vi "Read_Write_Temp_Cluster.vi"(3 "Template Info Array":T3[](array[typedef]) {"Tolerance" min=0.0 format="%#.4f"}, 4 "Mode":T2, 5 "Template File":path) -> (0 "Template Info Array Out":T3[](array[typedef]) {"Tolerance" min=0.0 format="%#.4f"})   [LabVIEW 2016]
uses:
  File_Template_Clus.ctl
  Data plotting/subVIs/Dispose_Channel.ctl
  Controls/Global_mode.ctl
panel:
  in  "Dispose":T1
  # "> 20  or  <20  or  =hello   or \n£hello  (not equal to hello)"
  # "<<Characters_to_Match>>  <<Replace_Whole_String_with_this>>"
  # "<<Channel_Name>> contains <<Characters to match>> or\n<<Channel_Name>> does not contain <<Characters to match>>"
  # "<<Channel_Name_A>> + <<Channel_Name_B>> or\nConcatenate <<Channel_Name_A>> and <<Channel_Name_B>>"
  # "> 20  or  <20  or  =hello   or \n£hello  (not equal to hello)"
  # "<<Characters_to_Match>>  <<Replace_Whole_String_with_this>>"
  # "<<Channel_Name>> contains <<Characters to match>> or\n<<Channel_Name>> does not contain <<Characters to match>>"
  # "<<Channel_Name_A>> + <<Channel_Name_B>> or\nConcatenate <<Channel_Name_A>> and <<Channel_Name_B>>"
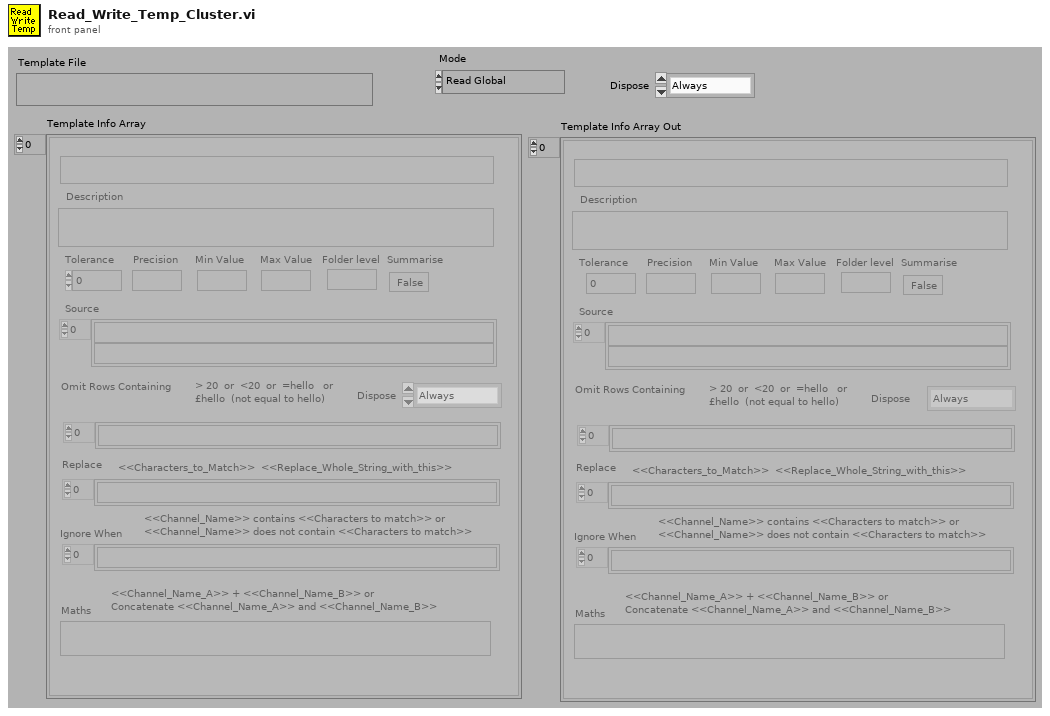
[diagram p1: front panel]
types:
  T1 = typedef "Dispose_Channel.ctl" = enum16{"Always", "If Blank", "Never"}
  T2 = typedef "Global_mode.ctl" = enum16{"Read Global", "Load Global From File", "Write Global to File"}
  T3 = typedef "File_Template_Clus.ctl" = cluster{"Template Channel Name":string, "Description":string, "Tolerance":dbl, "Precision":string, "Folder level":string, "Source":string[], "Replace":string[], "Summarise":bool, "Min Value":string, "Maths":string, "Omit Rows Containing":string[], "Ignore When":string[], "Max Value":string, "Dispose":T1}
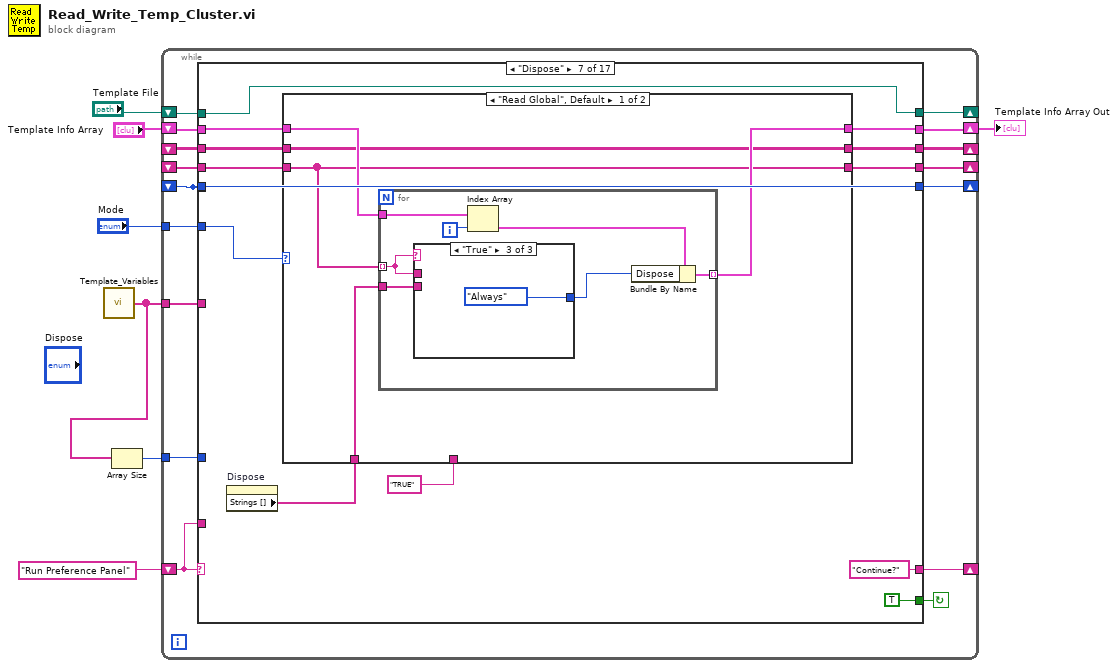
[diagram p0: block diagram]
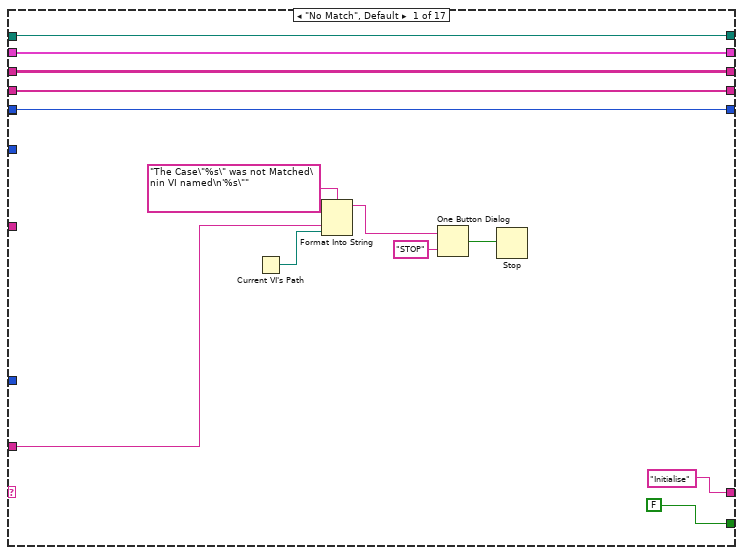
[diagram p2: hidden frame]
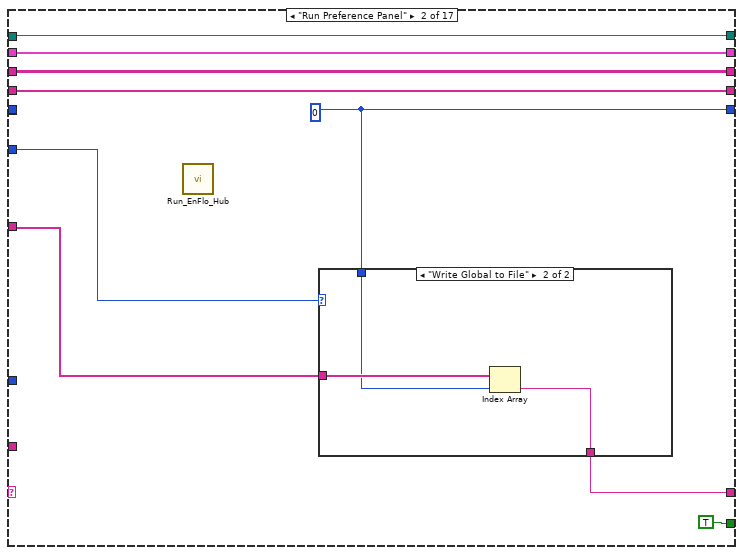
[diagram p3: hidden frame]
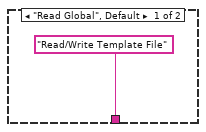
[diagram p4: hidden frame]
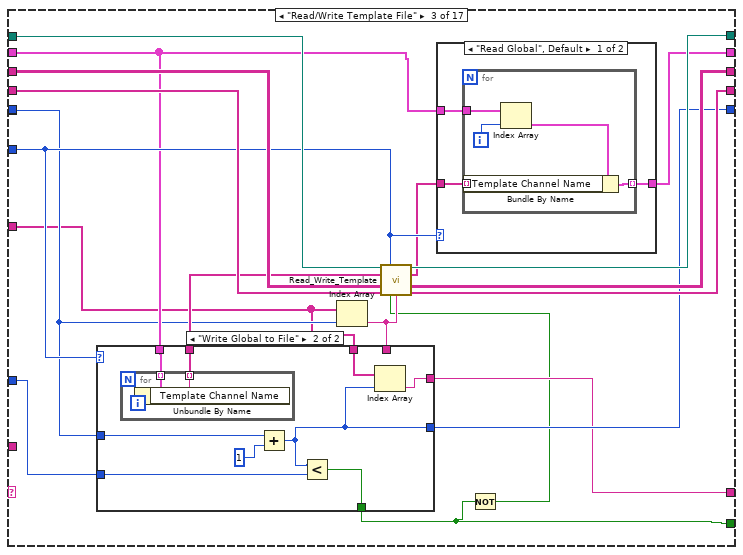
[diagram p5: hidden frame]
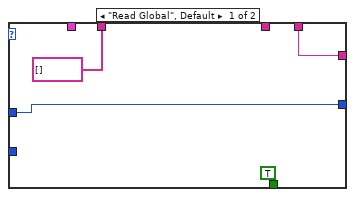
[diagram p7: hidden frame]
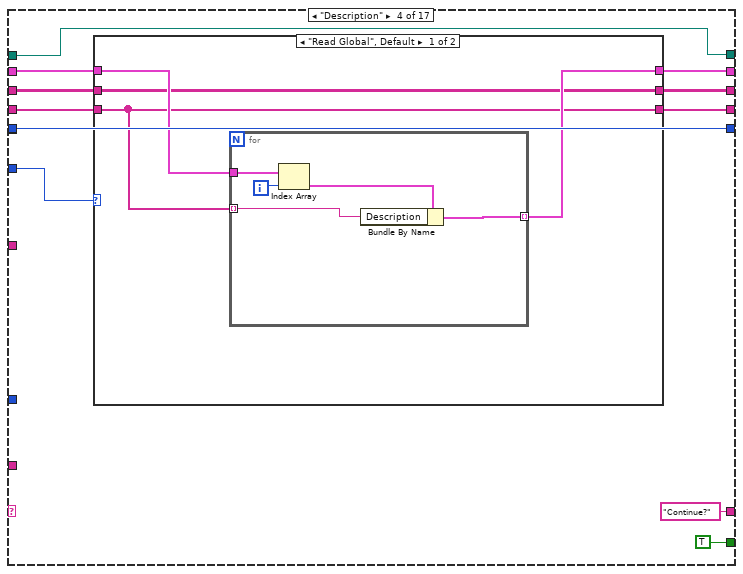
[diagram p8: hidden frame]
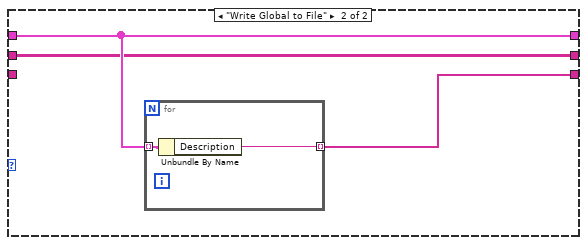
[diagram p9: hidden frame]
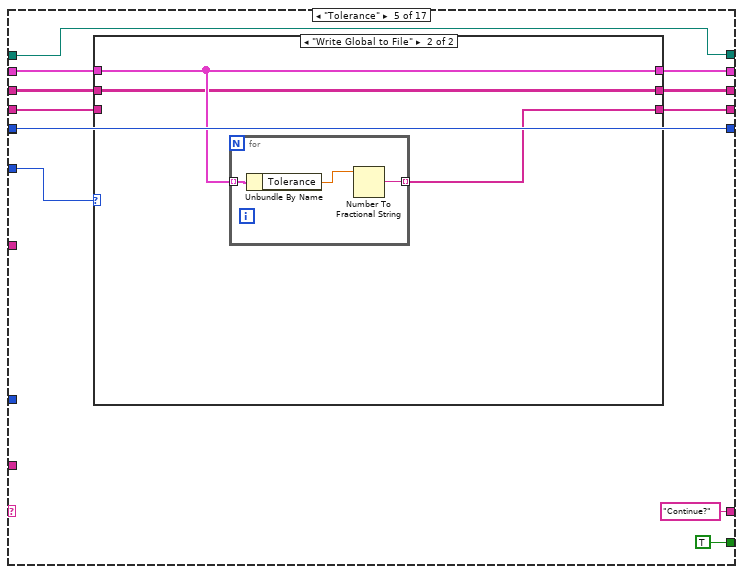
[diagram p10: hidden frame]
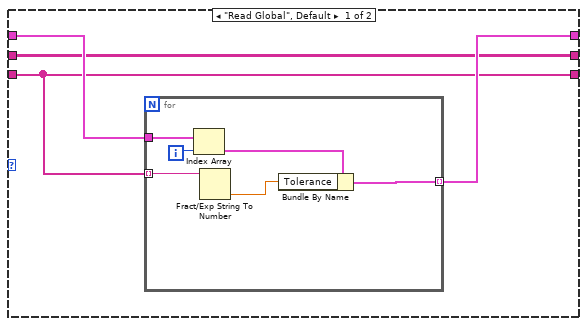
[diagram p11: hidden frame]
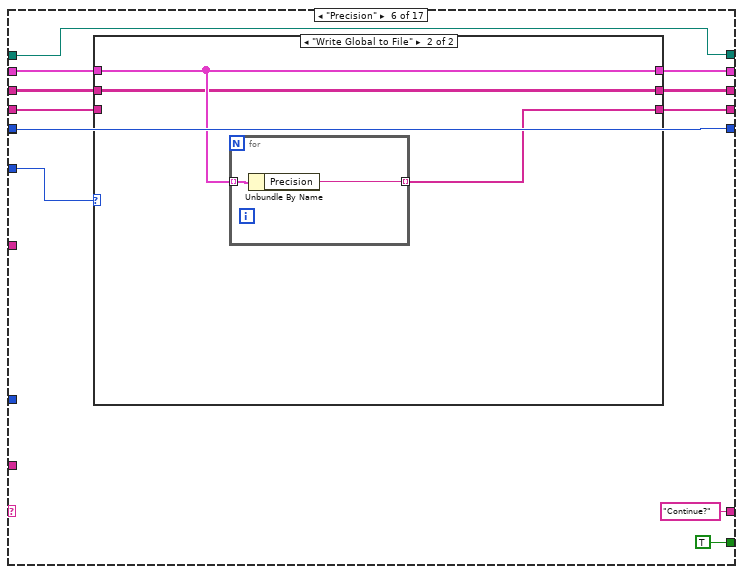
[diagram p12: hidden frame]
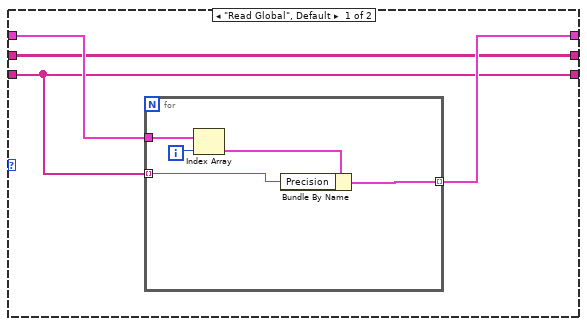
[diagram p13: hidden frame]
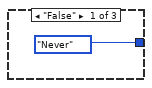
[diagram p14: hidden frame]
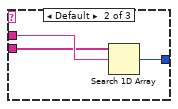
[diagram p15: hidden frame]
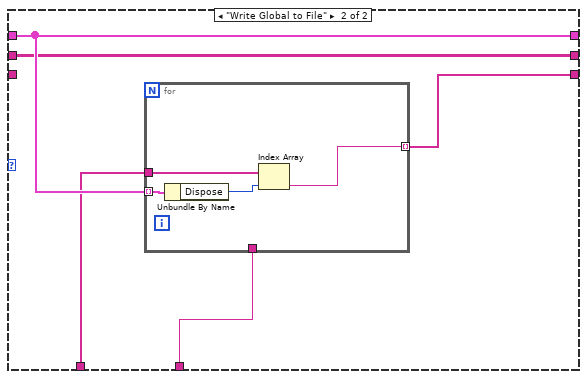
[diagram p16: hidden frame]
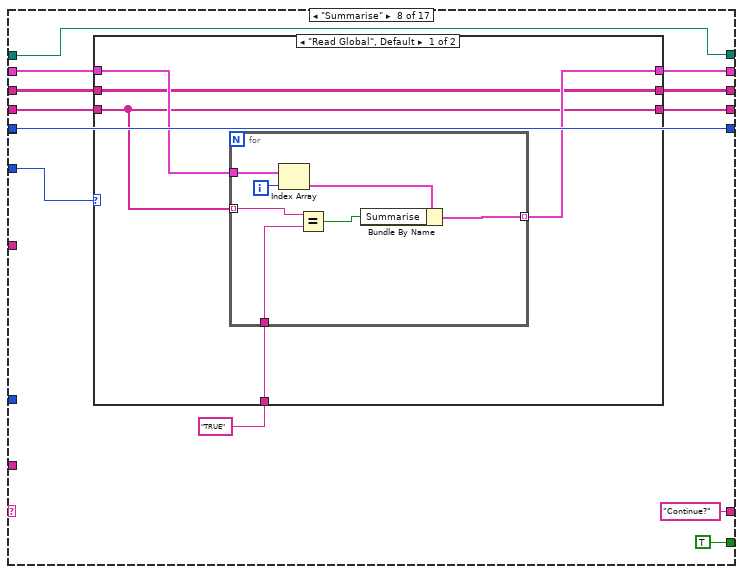
[diagram p17: hidden frame]
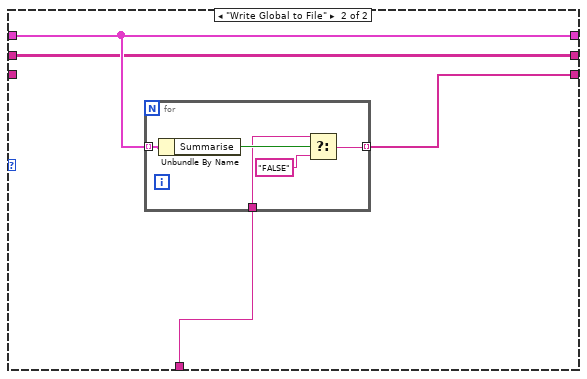
[diagram p18: hidden frame]
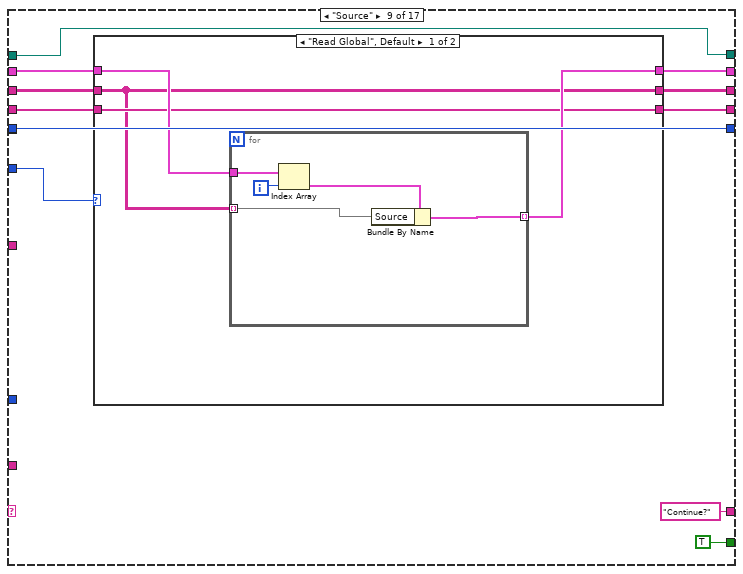
[diagram p19: hidden frame]
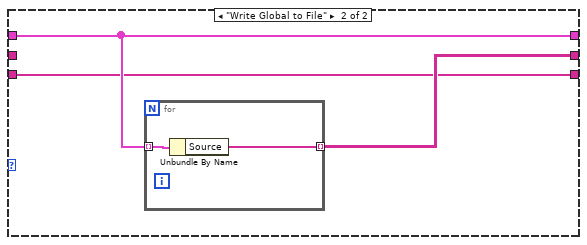
[diagram p20: hidden frame]
diagram:
  n1 = call "Template_Variables.vi"() -> ("Variable Names"=w1:string[])
  n2 = Array Size(array=w1) -> (size(s)=w2:i32)
  n3 = while {
    tunnel: w2 -> [w11]
    tunnel: "Mode" -> [w13]
    tunnel: w1 -> [w16]
    shift-left: "Template File" -> [w17]
    shift-right: [w8] -> _
    shift-left: _ -> [w10]
    shift-right: [w9] -> _
    shift-left: _ -> [w14]
    shift-right: [w18] -> _
    shift-left: _ -> [w15]
    shift-right: [w12] -> _
    shift-left: "Template Info Array" -> [w19]
    shift-right: [w20] -> w4
    shift-left: "Run Preference Panel" -> [w21]
    shift-right: [w22] -> _
    stop <- w23 continue-if-true
    n4 = case shown="\"Dispose\"" w21 {
      tunnel: [FALSE TRUE w51 TRUE TRUE TRUE TRUE TRUE TRUE TRUE TRUE TRUE TRUE TRUE TRUE TRUE w444] -> w23
      tunnel: ["Initialise" w39 w53 "Continue?" "Continue?" "Continue?" "Continue?" "Continue?" "Continue?" "Continue?" "Continue?" "Continue?" "Continue?" "Continue?" "Continue?" "Continue?" "Read/Write Template File"] -> w22
      tunnel: w21 -> [w31 _ _ _ _ _ _ _ _ _ _ _ _ _ _ _ _]
      tunnel: [w24 w43 w59 w95 w120 w147 w174 w212 w244 w269 w294 w319 w344 w369 w394 w419 w450] -> w20
      tunnel: w19 -> [w24 w43 w58 w102 w127 w154 w181 w219 w251 w276 w301 w326 w351 w376 w401 w426 w450]
      tunnel: [w27 w42 w68 w99 w124 w151 w178 w216 w248 w273 w298 w323 w348 w373 w398 w423 w449] -> w12
      tunnel: [w26 w41 w67 w98 w123 w150 w177 w215 w247 w272 w297 w322 w347 w372 w397 w422 w448] -> w18
      tunnel: [w28 w44 w65 w103 w128 w155 w182 w220 w252 w277 w302 w327 w352 w377 w402 w427 w451] -> w8
      tunnel: w17 -> [w28 w44 w66 w103 w128 w155 w182 w220 w252 w277 w302 w327 w352 w377 w402 w427 w451]
      tunnel: w10 -> [w25 _ w56 w93 w118 w145 w171 w209 w242 w267 w292 w317 w342 _ w392 w417 w443]
      tunnel: w16 -> [_ w38 w54 _ _ _ _ _ _ _ _ _ _ _ _ _ w446]
      tunnel: w15 -> [w27 w42 w64 w100 w125 w152 w179 w217 w249 w274 w299 w324 w349 w374 w399 w424 w449]
      tunnel: w14 -> [w26 w41 w63 w101 w126 w153 w180 w218 w250 w275 w300 w325 w350 w375 w400 w425 w448]
      tunnel: w13 -> [_ w40 w60 w94 w119 w146 w172 w210 w243 w268 w293 w318 w343 w368 w393 w418 w447]
      tunnel: w11 -> [_ _ w62 _ _ _ _ _ _ _ _ _ _ _ _ _ _]
      tunnel: w10 -> [_ _ _ _ _ _ _ _ _ _ _ _ _ w367 _ _ _]
      tunnel: [w25 w37 w55 w93 w118 w145 w171 w209 w242 w267 w292 w317 w342 w367 w392 w417 w442] -> w9
      frame "No Match", Default {
        n5 = Current VI's Path() -> (path=w30:path)
        n6 = Format Into String(format string="The Case\"%s\" was not Matched\nin VI named\n'%s\"" ("Format String"), w31, w30) -> (resulting string=w34:string)  [unwired: 2 in, 1 out]
        n7 = One Button Dialog(message=w34, button name ("OK")="STOP") -> (true=w32:bool)
        n8 = Stop(stop? (T)=w32) -> ()
      }
      frame "Run Preference Panel" {
        w37 = 0
        n9 = call "Run_EnFlo_Hub.vi"() -> ()  [unwired: 1 in, 7 out]
        n10 = case shown="\"Write Global to File\"" w40 {
          tunnel: ["Read/Write Template File" w48] -> w39
          tunnel: w38 -> [_ w49]
          tunnel: w37 -> [_ w47]
          frame "Read Global", Default {
          }
          frame "Write Global to File" {
            n11 = Index Array(array=w49, index=w47) -> (element=w48:string)
          }
        }
      }
      frame "Read/Write Template File" {
        n12 = Index Array(array=w54, index=w56) -> (element=w52:string)
        n13 = case shown="\"Write Global to File\"" w60 {
          tunnel: [w79 w84] -> w55
          tunnel: w56 -> [w79 w89]
          tunnel: w62 -> [_ w88]
          tunnel: [TRUE w87] -> w51
          tunnel: w58 -> [_ w86]
          tunnel: [string[] [] w85] -> w61
          tunnel: w54 -> [_ w83]
          tunnel: [w78 w82] -> w53
          tunnel: w52 -> [w78 _]
          frame "Read Global", Default {
          }
          frame "Write Global to File" {
            n14 = for {
              tunnel: w86 -> [w92] mode=indexing
              tunnel: [w91] -> w85 mode=indexing
              n15 = Unbundle By Name(w92) -> ("Template Channel Name"=w91:string)
            }
            n16 = Add(x=w89, y=1) -> (x+y=w84:i32)
            n17 = Less?(x=w84, y=w88) -> (x < y?=w87:bool)
            n18 = Index Array(array=w83, index=w84) -> (element=w82:string)
          }
        }
        n19 = Not(x=w51) -> (.not. x?=w50:bool)
        n20 = call "Read_Write_Template.vi"("Template File"=w66, "Mode"=w60, "Channel names In"=w61, "2D Info In"=w64, "1D Info In"=w63, "Save file"=w50, "Data type"=w52) -> ("Template File Out"=w65:path, "Template Ch Names Out"=w57:string[], "2D Info Out"=w68:string[][], "1D Info Out"=w67:string[])  [unwired: 1 in, 4 out]
        n21 = case shown="\"Read Global\", Default" w60 {
          tunnel: w58 -> [w71 w77]
          tunnel: [w70 w77] -> w59
          tunnel: w57 -> [w69 _]
          frame "Read Global", Default {
            n22 = for {
              tunnel: w71 -> [w74]
              tunnel: [w76] -> w70 mode=indexing
              tunnel: w69 -> [w75] mode=indexing
              i -> [w73]
              n23 = Index Array(array=w74, index=w73) -> (element=w72:T3)
              n24 = Bundle By Name(cluster=w72, "Template Channel Name"=w75) -> (w76:T3)
            }
          }
          frame "Write Global to File" {
          }
        }
      }
      frame "Description" {
        n25 = case shown="\"Read Global\", Default" w94 {
          tunnel: w102 -> [w107 w115]
          tunnel: w101 -> [w104 _]
          tunnel: [w106 w115] -> w95
          tunnel: w100 -> [w105 w113]
          tunnel: [w105 w113] -> w99
          tunnel: [w104 w114] -> w98
          frame "Read Global", Default {
            n26 = for {
              tunnel: w107 -> [w111]
              tunnel: w104 -> [w108] mode=indexing
              tunnel: [w109] -> w106 mode=indexing
              i -> [w112]
              n27 = Index Array(array=w111, index=w112) -> (element=w110:T3)
              n28 = Bundle By Name(cluster=w110, "Description"=w108) -> (w109:T3)
            }
          }
          frame "Write Global to File" {
            n29 = for {
              tunnel: w115 -> [w117] mode=indexing
              tunnel: [w116] -> w114 mode=indexing
              n30 = Unbundle By Name(w117) -> ("Description"=w116:string)
            }
          }
        }
      }
      frame "Tolerance" {
        n31 = case shown="\"Write Global to File\"" w119 {
          tunnel: w127 -> [w132 w141]
          tunnel: w126 -> [w129 _]
          tunnel: [w131 w141] -> w120
          tunnel: w125 -> [w130 w139]
          tunnel: [w130 w139] -> w124
          tunnel: [w129 w140] -> w123
          frame "Read Global", Default {
            n32 = for {
              tunnel: w132 -> [w137]
              tunnel: w129 -> [w135] mode=indexing
              tunnel: [w133] -> w131 mode=indexing
              i -> [w138]
              n33 = Index Array(array=w137, index=w138) -> (element=w136:T3)
              n34 = Fract/Exp String To Number(string=w135) -> (number=w134:dbl)  [unwired: 4 out]
              n35 = Bundle By Name(cluster=w136, "Tolerance"=w134) -> (w133:T3)
            }
          }
          frame "Write Global to File" {
            n36 = for {
              tunnel: w141 -> [w144] mode=indexing
              tunnel: [w142] -> w140 mode=indexing
              n37 = Unbundle By Name(w144) -> ("Tolerance"=w143:dbl)
              n38 = Number To Fractional String(number=w143) -> (F-format string=w142:string)  [unwired: 3 out]
            }
          }
        }
      }
      frame "Precision" {
        n39 = case shown="\"Write Global to File\"" w146 {
          tunnel: w154 -> [w159 w167]
          tunnel: w153 -> [w156 _]
          tunnel: [w158 w167] -> w147
          tunnel: w152 -> [w157 w165]
          tunnel: [w157 w165] -> w151
          tunnel: [w156 w166] -> w150
          frame "Read Global", Default {
            n40 = for {
              tunnel: w159 -> [w163]
              tunnel: w156 -> [w160] mode=indexing
              tunnel: [w161] -> w158 mode=indexing
              i -> [w164]
              n41 = Index Array(array=w163, index=w164) -> (element=w162:T3)
              n42 = Bundle By Name(cluster=w162, "Precision"=w160) -> (w161:T3)
            }
          }
          frame "Write Global to File" {
            n43 = for {
              tunnel: w167 -> [w169] mode=indexing
              tunnel: [w168] -> w166 mode=indexing
              n44 = Unbundle By Name(w169) -> ("Precision"=w168:string)
            }
          }
        }
      }
      frame "Dispose" {
        n45 = property on="Dispose" class="Enum (strict)"() -> ("Strings []"=w170:string[])  [unwired: 2 in, 2 out]
        n46 = case shown="\"Read Global\", Default" w172 {
          tunnel: w181 -> [w187 w204]
          tunnel: w180 -> [w184 _]
          tunnel: [w186 w204] -> w174
          tunnel: w179 -> [w185 w202]
          tunnel: [w185 w202] -> w178
          tunnel: [w184 w203] -> w177
          tunnel: "TRUE" ("y") -> [_ w201]
          tunnel: w170 -> [w183 w200]
          frame "Read Global", Default {
            n47 = for {
              tunnel: w187 -> [w193]
              tunnel: w184 -> [w188] mode=indexing
              tunnel: [w191] -> w186 mode=indexing
              tunnel: w183 -> [w190]
              i -> [w194]
              n48 = case shown="\"True\"" w188 {
                tunnel: w188 -> [_ w198 _]
                tunnel: w190 -> [_ w197 _]
                tunnel: [Dispose_Channel."Never" ("Dispose") w196 Dispose_Channel."Always" ("Dispose")] -> w189
                frame "False" {
                }
                frame Default {
                  n49 = Search 1D Array(1D array=w197, element=w198) -> (index of element=w196:i32)  [unwired: 1 in]
                }
                frame "True" {
                }
              }
              n50 = Index Array(array=w193, index=w194) -> (element=w192:T3)
              n51 = Bundle By Name(cluster=w192, "Dispose"=w189) -> (w191:T3)
            }
          }
          frame "Write Global to File" {
            n52 = for {
              tunnel: w204 -> [w208] mode=indexing
              tunnel: [w205] -> w203 mode=indexing
              tunnel: w201 -> [_]
              tunnel: w200 -> [w206]
              n53 = Unbundle By Name(w208) -> ("Dispose"=w207:T1)
              n54 = Index Array(array=w206, index=w207) -> (element=w205:string)
            }
          }
        }
      }
      frame "Summarise" {
        n55 = case shown="\"Read Global\", Default" w210 {
          tunnel: w219 -> [w225 w236]
          tunnel: w218 -> [w222 _]
          tunnel: [w224 w236] -> w212
          tunnel: w217 -> [w223 w234]
          tunnel: [w223 w234] -> w216
          tunnel: [w222 w235] -> w215
          tunnel: "TRUE" ("y") -> [w221 w233]
          frame "Read Global", Default {
            n56 = for {
              tunnel: w225 -> [w231]
              tunnel: w222 -> [w228] mode=indexing
              tunnel: [w229] -> w224 mode=indexing
              tunnel: w221 -> [w226]
              i -> [w232]
              n57 = Index Array(array=w231, index=w232) -> (element=w230:T3)
              n58 = Equal?(x=w228, y=w226) -> (x = y?=w227:bool)
              n59 = Bundle By Name(cluster=w230, "Summarise"=w227) -> (w229:T3)
            }
          }
          frame "Write Global to File" {
            n60 = for {
              tunnel: w236 -> [w241] mode=indexing
              tunnel: [w237] -> w235 mode=indexing
              tunnel: w233 -> [w239]
              n61 = Unbundle By Name(w241) -> ("Summarise"=w240:bool)
              n62 = Select(t=w239, s=w240, f="FALSE") -> (s? t:f=w237:string)
            }
          }
        }
      }
      frame "Source" {
        n63 = case shown="\"Read Global\", Default" w243 {
          tunnel: w251 -> [w256 w264]
          tunnel: w250 -> [w254 w262]
          tunnel: [w255 w264] -> w244
          tunnel: w249 -> [w253 _]
          tunnel: [w253 w263] -> w248
          tunnel: [w254 w262] -> w247
          frame "Read Global", Default {
            n64 = for {
              tunnel: w256 -> [w260]
              tunnel: w253 -> [w257] mode=indexing
              tunnel: [w258] -> w255 mode=indexing
              i -> [w261]
              n65 = Index Array(array=w260, index=w261) -> (element=w259:T3)
              n66 = Bundle By Name(cluster=w259, "Source"=w257) -> (w258:T3)
            }
          }
          frame "Write Global to File" {
            n67 = for {
              tunnel: w264 -> [w266] mode=indexing
              tunnel: [w265] -> w263 mode=indexing
              n68 = Unbundle By Name(w266) -> ("Source"=w265:string[])
            }
          }
        }
      }
      frame "Ignore When" {
        n69 = case shown="\"Read Global\", Default" w268 {
          tunnel: w276 -> [w281 w289]
          tunnel: w275 -> [w279 w287]
          tunnel: [w280 w289] -> w269
          tunnel: w274 -> [w278 _]
          tunnel: [w278 w288] -> w273
          tunnel: [w279 w287] -> w272
          frame "Read Global", Default {
            n70 = for {
              tunnel: w281 -> [w285]
              tunnel: w278 -> [w282] mode=indexing
              tunnel: [w283] -> w280 mode=indexing
              i -> [w286]
              n71 = Index Array(array=w285, index=w286) -> (element=w284:T3)
              n72 = Bundle By Name(cluster=w284, "Ignore When"=w282) -> (w283:T3)
            }
          }
          frame "Write Global to File" {
            n73 = for {
              tunnel: w289 -> [w291] mode=indexing
              tunnel: [w290] -> w288 mode=indexing
              n74 = Unbundle By Name(w291) -> ("Ignore When"=w290:string[])
            }
          }
        }
      }
      frame "Replace" {
        n75 = case shown="\"Read Global\", Default" w293 {
          tunnel: w301 -> [w306 w314]
          tunnel: w300 -> [w304 w312]
          tunnel: [w305 w314] -> w294
          tunnel: w299 -> [w303 _]
          tunnel: [w303 w313] -> w298
          tunnel: [w304 w312] -> w297
          frame "Read Global", Default {
            n76 = for {
              tunnel: w306 -> [w310]
              tunnel: w303 -> [w307] mode=indexing
              tunnel: [w308] -> w305 mode=indexing
              i -> [w311]
              n77 = Index Array(array=w310, index=w311) -> (element=w309:T3)
              n78 = Bundle By Name(cluster=w309, "Replace"=w307) -> (w308:T3)
            }
          }
          frame "Write Global to File" {
            n79 = for {
              tunnel: w314 -> [w316] mode=indexing
              tunnel: [w315] -> w313 mode=indexing
              n80 = Unbundle By Name(w316) -> ("Replace"=w315:string[])
            }
          }
        }
      }
      frame "Maths" {
        n81 = case shown="\"Read Global\", Default" w318 {
          tunnel: w326 -> [w331 w339]
          tunnel: w325 -> [w328 _]
          tunnel: [w330 w339] -> w319
          tunnel: w324 -> [w329 w337]
          tunnel: [w329 w337] -> w323
          tunnel: [w328 w338] -> w322
          frame "Read Global", Default {
            n82 = for {
              tunnel: w331 -> [w335]
              tunnel: w328 -> [w332] mode=indexing
              tunnel: [w333] -> w330 mode=indexing
              i -> [w336]
              n83 = Index Array(array=w335, index=w336) -> (element=w334:T3)
              n84 = Bundle By Name(cluster=w334, "Maths"=w332) -> (w333:T3)
            }
          }
          frame "Write Global to File" {
            n85 = for {
              tunnel: w339 -> [w341] mode=indexing
              tunnel: [w340] -> w338 mode=indexing
              n86 = Unbundle By Name(w341) -> ("Maths"=w340:string)
            }
          }
        }
      }
      frame "Omit" {
        n87 = case shown="\"Write Global to File\"" w343 {
          tunnel: w351 -> [w356 w364]
          tunnel: w350 -> [w354 w362]
          tunnel: [w355 w364] -> w344
          tunnel: w349 -> [w353 _]
          tunnel: [w353 w363] -> w348
          tunnel: [w354 w362] -> w347
          frame "Read Global", Default {
            n88 = for {
              tunnel: w356 -> [w360]
              tunnel: w353 -> [w357] mode=indexing
              tunnel: [w358] -> w355 mode=indexing
              i -> [w361]
              n89 = Index Array(array=w360, index=w361) -> (element=w359:T3)
              n90 = Bundle By Name(cluster=w359, "Omit Rows Containing"=w357) -> (w358:T3)
            }
          }
          frame "Write Global to File" {
            n91 = for {
              tunnel: w364 -> [w366] mode=indexing
              tunnel: [w365] -> w363 mode=indexing
              n92 = Unbundle By Name(w366) -> ("Omit Rows Containing"=w365:string[])
            }
          }
        }
      }
      frame "Folder level" {
        n93 = case shown="\"Write Global to File\"" w368 {
          tunnel: w376 -> [w381 w389]
          tunnel: w375 -> [w378 _]
          tunnel: [w380 w389] -> w369
          tunnel: w374 -> [w379 w387]
          tunnel: [w379 w387] -> w373
          tunnel: [w378 w388] -> w372
          frame "Read Global", Default {
            n94 = for {
              tunnel: w381 -> [w385]
              tunnel: w378 -> [w382] mode=indexing
              tunnel: [w383] -> w380 mode=indexing
              i -> [w386]
              n95 = Index Array(array=w385, index=w386) -> (element=w384:T3)
              n96 = Bundle By Name(cluster=w384, "Folder level"=w382) -> (w383:T3)
            }
          }
          frame "Write Global to File" {
            n97 = for {
              tunnel: w389 -> [w391] mode=indexing
              tunnel: [w390] -> w388 mode=indexing
              n98 = Unbundle By Name(w391) -> ("Folder level"=w390:string)
            }
          }
        }
      }
      frame "Minimum Value" {
        n99 = case shown="\"Write Global to File\"" w393 {
          tunnel: w401 -> [w406 w414]
          tunnel: w400 -> [w403 _]
          tunnel: [w405 w414] -> w394
          tunnel: w399 -> [w404 w412]
          tunnel: [w404 w412] -> w398
          tunnel: [w403 w413] -> w397
          frame "Read Global", Default {
            n100 = for {
              tunnel: w406 -> [w410]
              tunnel: w403 -> [w408] mode=indexing
              tunnel: [w407] -> w405 mode=indexing
              i -> [w411]
              n101 = Index Array(array=w410, index=w411) -> (element=w409:T3)
              n102 = Bundle By Name(cluster=w409, "Min Value"=w408) -> (w407:T3)
            }
          }
          frame "Write Global to File" {
            n103 = for {
              tunnel: w414 -> [w416] mode=indexing
              tunnel: [w415] -> w413 mode=indexing
              n104 = Unbundle By Name(w416) -> ("Min Value"=w415:string)
            }
          }
        }
      }
      frame "Maximum Value" {
        n105 = case shown="\"Read Global\", Default" w418 {
          tunnel: w426 -> [w431 w439]
          tunnel: w425 -> [w428 _]
          tunnel: [w430 w439] -> w419
          tunnel: w424 -> [w429 w437]
          tunnel: [w429 w437] -> w423
          tunnel: [w428 w438] -> w422
          frame "Read Global", Default {
            n106 = for {
              tunnel: w431 -> [w435]
              tunnel: w428 -> [w433] mode=indexing
              tunnel: [w432] -> w430 mode=indexing
              i -> [w436]
              n107 = Index Array(array=w435, index=w436) -> (element=w434:T3)
              n108 = Bundle By Name(cluster=w434, "Max Value"=w433) -> (w432:T3)
            }
          }
          frame "Write Global to File" {
            n109 = for {
              tunnel: w439 -> [w441] mode=indexing
              tunnel: [w440] -> w438 mode=indexing
              n110 = Unbundle By Name(w441) -> ("Max Value"=w440:string)
            }
          }
        }
      }
      frame "Continue?" {
        n111 = Array Size(array=w446) -> (size(s)=w445:i32)
        n112 = case shown="\"Read Global\", Default" w447 {
          tunnel: w445 -> [w457 _]
          tunnel: [w456 TRUE] -> w444
          tunnel: w443 -> [w454 w458]
          tunnel: [w453 w458] -> w442
          frame "Read Global", Default {
            n113 = Add(x=w454, y=1) -> (x+y=w453:i32)
            n114 = Less?(x=w453, y=w457) -> (x < y?=w456:bool)
          }
          frame "Write Global to File" {
          }
        }
      }
    }
  }
  "Template Info Array Out" <- w4
